vi "set_plot_axis_data.vi"(9 "plot_allocation":T1(array[cluster]), 10 "plot_data":cluster{"freq_array_out":dbl[], dbl[]}[](array[cluster]), 11 "reference":refnum<vi>) -> (0 "done":bool)   [LabVIEW 2025]
panel:
  # "[plot_id], [data_id], [y_scale/unit]"
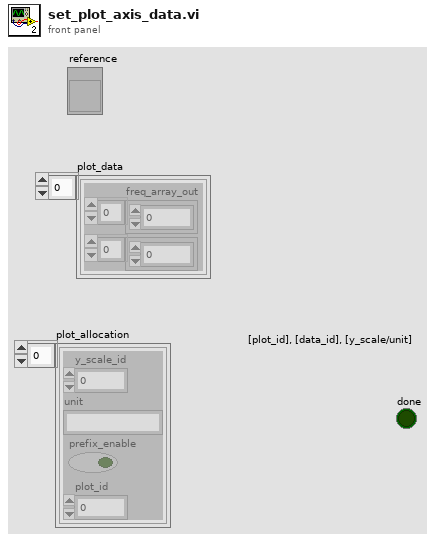
[diagram p1: front panel]
types:
  T1 = cluster{"y_scale_id":u32, "unit":string, "prefix_enable":bool, "plot_id":u32}[]
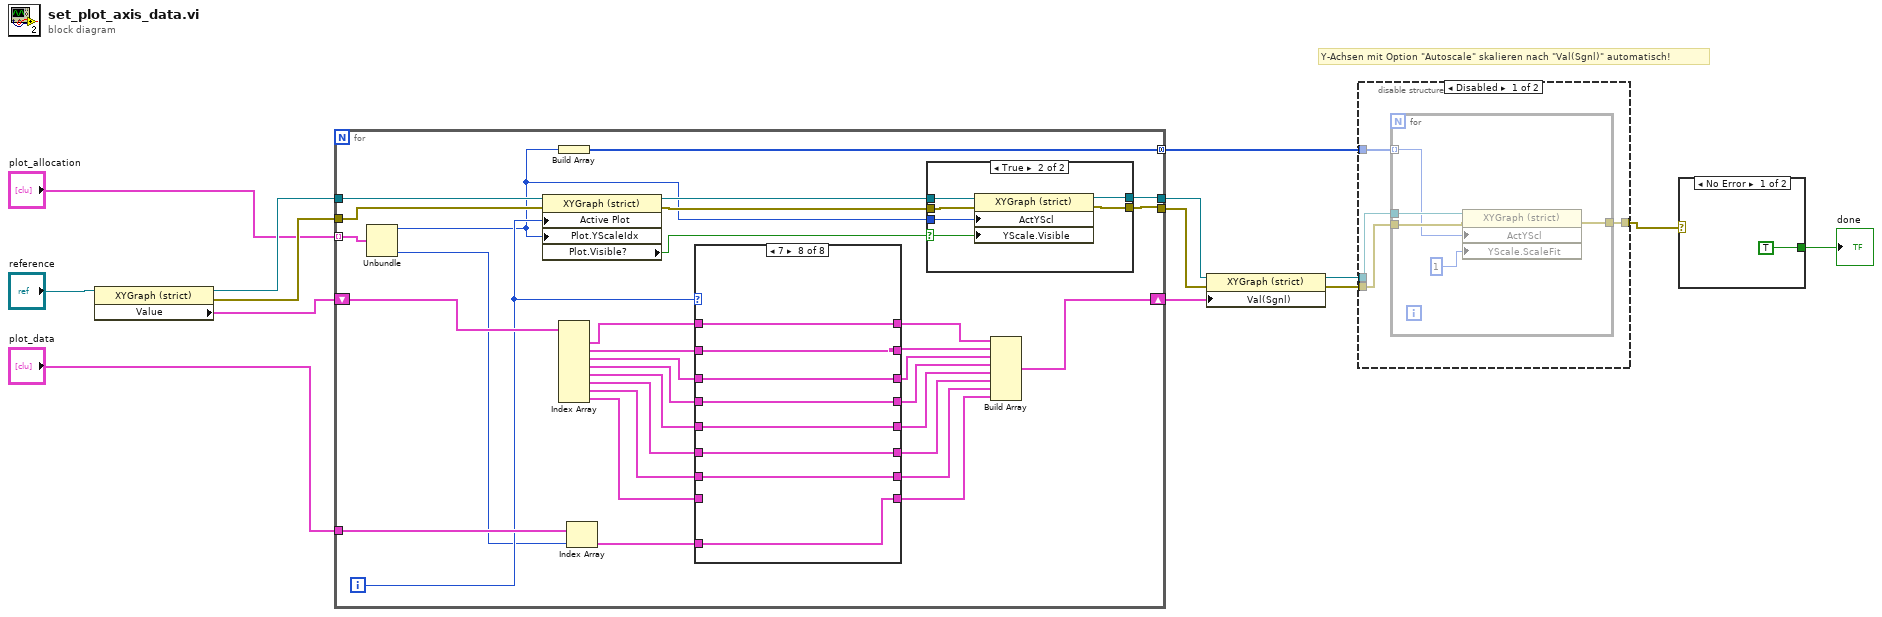
[diagram p0: block diagram]
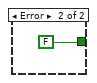
[diagram p3: hidden frame]
diagram:
  # "Y-Achsen mit Option \"Autoscale\" skalieren nach \"Val(Sgnl)\" automatisch!"
  n1 = property on="Property Node" class="XYGraph (strict)"(reference="reference") -> (reference out=w9:refnum<vi>, error out=w7:errorcluster, "Value"=w11:cluster{"array type (2D Dbl)":dbl[], dbl[]}[])  [unwired: 1 in]
  n2 = for {
    tunnel: "plot_data" -> [w45]
    shift-right: [w46] -> w14
    shift-left: w11 -> [w27]
    tunnel: "plot_allocation" -> [w25] mode=indexing
    tunnel: w9 -> [w26]
    tunnel: [w20] -> w13
    tunnel: w7 -> [w24]
    tunnel: [w19] -> w8
    tunnel: [w18] -> w3 mode=concatenating
    i -> [w17]
    n3 = Unbundle(w25) -> ("y_scale_id"=w15:u32, "plot_id"=w16:u32)  [unwired: 2 out]
    n4 = property on="Property Node" class="XYGraph (strict)"(reference=w26, error in=w24, "Active Plot"=w17, "Plot.YScaleIdx"=w15) -> (reference out=w23:refnum<vi>, error out=w22:errorcluster, "Plot.Visible?"=w21:bool)
    n5 = Build Array(w15) -> (w18:u32[])
    n6 = Index Array(array=w27) -> (element #1=w38:cluster{"array type (2D Dbl)":dbl[], dbl[]}, element #2=w41:cluster{"array type (2D Dbl)":dbl[], dbl[]}, element #3=w39:cluster{"array type (2D Dbl)":dbl[], dbl[]}, element #4=w36:cluster{"array type (2D Dbl)":dbl[], dbl[]}, element #5=w34:cluster{"array type (2D Dbl)":dbl[], dbl[]}, element #6=w32:cluster{"array type (2D Dbl)":dbl[], dbl[]}, element #7=w30:cluster{"array type (2D Dbl)":dbl[], dbl[]}, element #8=w28:cluster{"array type (2D Dbl)":dbl[], dbl[]})  [unwired: 8 in]
    n7 = Index Array(array=w45, index=w16) -> (element=w43:cluster{"freq_array_out":dbl[], dbl[]})
    n8 = case shown="7" w17 {
      tunnel: [w62 w69 w76 w85 w93 w101 w109 w117] -> w44
      tunnel: w43 -> [w62 w70 w78 w80 w88 w96 w104 w112]
      tunnel: [w61 w70 w77 w86 w94 w102 w110 w118] -> w42
      tunnel: w41 -> [w61 _ w77 w86 w94 w102 w110 w118]
      tunnel: [w60 w68 w78 w79 w89 w98 w107 w116] -> w40
      tunnel: w39 -> [w60 w68 _ w79 w89 w98 w107 w116]
      tunnel: w38 -> [_ w69 w76 w85 w93 w101 w109 w117]
      tunnel: [w59 w67 w75 w80 w87 w97 w106 w115] -> w37
      tunnel: w36 -> [w59 w67 w75 _ w87 w97 w106 w115]
      tunnel: [w58 w66 w74 w84 w88 w95 w105 w114] -> w35
      tunnel: w34 -> [w58 w66 w74 w84 _ w95 w105 w114]
      tunnel: [w57 w65 w73 w83 w92 w96 w103 w113] -> w33
      tunnel: w32 -> [w57 w65 w73 w83 w92 _ w103 w113]
      tunnel: [w56 w64 w72 w82 w91 w100 w104 w111] -> w31
      tunnel: w30 -> [w56 w64 w72 w82 w91 w100 _ w111]
      tunnel: [w55 w63 w71 w81 w90 w99 w108 w112] -> w29
      tunnel: w28 -> [w55 w63 w71 w81 w90 w99 w108 _]
      frame 0, Default {
      }
      frame 1 {
      }
      frame 2 {
      }
      frame 3 {
      }
      frame 4 {
      }
      frame 5 {
      }
      frame 6 {
      }
      frame 7 {
      }
    }
    n9 = case shown="True" w21 {
      selector: w21 -> [_ w52]
      tunnel: w23 -> [w48 w54]
      tunnel: w22 -> [w47 w53]
      tunnel: w15 -> [_ w51]
      tunnel: [w48 w50] -> w20
      tunnel: [w47 w49] -> w19
      frame False {
      }
      frame True {
        n10 = property on="Property Node" class="XYGraph (strict)"(reference=w54, error in=w53, "ActYScl"=w51, "YScale.Visible"=w52) -> (reference out=w50:refnum<vi>, error out=w49:errorcluster)
      }
    }
    n11 = Build Array(w44, w42, w40, w37, w35, w33, w31, w29) -> (w46:cluster{"freq_array_out":dbl[], dbl[]}[])
  }
  n12 = property on="Property Node" class="XYGraph (strict)"(reference=w13, error in=w8, "Val(Sgnl)"=w14) -> (reference out=w5:refnum<vi>, error out=w4:errorcluster)
  n13 = disable-structure shown="Disabled" {
    disable-tunnel: w5 -> [w122 _]
    disable-tunnel: w4 -> [w121 w128]
    disable-tunnel: w3 -> [w120 _]
    disable-tunnel: [w119 w128] -> w2
    frame Disabled {
      n14 = for {
        tunnel: w122 -> [w126]
        tunnel: w121 -> [w125]
        tunnel: w120 -> [w124] mode=indexing
        tunnel: [w123] -> w119
        n15 = property on="Property Node" class="XYGraph (strict)"(reference=w126, error in=w125, "ActYScl"=w124, "YScale.ScaleFit"=u8 1 ("Y Scale.Scale Fit")) -> (error out=w123:errorcluster)  [unwired: 1 out]
      }
    }
    frame Enabled {
    }
  }
  n16 = case shown="No Error" w2 {
    tunnel: [TRUE FALSE] -> w6
    frame No Error {
    }
    frame Error {
    }
  }
  "done" <- w6
